vi "closetiffs.vi"   [LabVIEW 2015]
types:
  T1 = typedef "LVRectTypeDef.ctl" = cluster{"Left":i16, "Top":i16, "Right":i16, "Bottom":i16}
  T2 = cluster{"Xpixels":i32, "Vxminref":dbl, "Vxmaxref":dbl, "P":dbl, "Ypixels":i32, "Vyminref":dbl, "Vymaxref":dbl, "srate":sgl, "sAOxy":i32, "timeout":dbl, "type":string, "date":string, "time":string, "Colormap":u16, "Drawing Mode":u16, "Scanning Mode":u16, "square pixels":bool, "square matrix":bool, "Xpixels Img":i32, "Vx-min Img":dbl, "VX-max Img":dbl, "Ypixels Img":i32, "Vy-min Img":dbl, "Vy-max Img ":dbl, "Angle Img":dbl, "autoshutter":bool, "finite":bool, "cont":bool, "wavdet":bool, "measpoints":i32, "avpp":i32, "bufferAO":i32, "bufferAI":i32, "starttick":u32, "waveform":path, "Vx-ref":dbl, "Vy-ref":dbl, "refreshrate":dbl, "refreshbuffer":i32, "tt_cycles":i32, "motorref":refnum<k7>, "mirrorswitch":refnum<k7>, "sample mode":i32, "maxbufferAI":i32, "srateAODO":sgl, "bin":sgl, "Pel":sgl, "Angle draw":dbl, "srate Img":sgl, "ROIimg_plotbounds":T1, "auto OD":bool, "ODfilt":u16, "aAI":i32[], "aCI":i32[], "aAO":u32[], "aDO":u32[], "refwfsize":dbl, "Lifetime":bool, "Vz-Img":dbl, "Vz-ref":dbl, "Vz-reset":dbl, "AIoverride":bool, "aAS":u32[], "XYZstart":dbl[], "External 100KHz Clock?":bool}
  T3 = cluster{"filetif":refnum<file>[], "E_filetif":errorcluster[]}
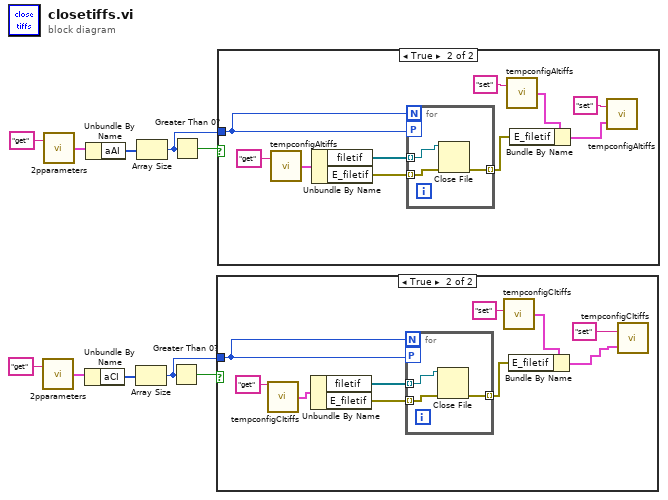
[diagram p0: block diagram]
diagram:
  n1 = call "2pparameters.vi"("command"="get") -> ("params out"=w1:T2)  [unwired: 1 in]
  n2 = call "2pparameters.vi"("command"="get") -> ("params out"=w10:T2)  [unwired: 1 in]
  n3 = Unbundle By Name(w1) -> ("aCI"=w3:i32[])
  n4 = Unbundle By Name(w10) -> ("aAI"=w8:i32[])
  n5 = Array Size(array=w3) -> (size(s)=w5:i32)
  n6 = Array Size(array=w8) -> (size(s)=w6:i32)
  n7 = Greater Than 0?(x=w5) -> (x > 0?=w4:bool)
  n8 = Greater Than 0?(x=w6) -> (x > 0?=w7:bool)
  n9 = case shown="True" w4 {
    tunnel: w5 -> [_ w17]
    frame False {
    }
    frame True {
      n10 = call "tempconfigCItiffs.vi"("command"="get") -> ("Temp Config out"=w15:T3)  [unwired: 1 in]
      n11 = Unbundle By Name(w15) -> ("filetif"=w20:refnum<file>[], "E_filetif"=w19:errorcluster[])
      n12 = for {
        N: w17 -> [_]
        workers-P: w17 -> [_]
        tunnel: w20 -> [w23] mode=indexing
        tunnel: w19 -> [w22] mode=indexing
        tunnel: [w21] -> w18 mode=indexing
        n13 = Close File(refnum=w23, error in=w22) -> (error out=w21:errorcluster)  [unwired: 1 out]
      }
      n14 = call "tempconfigCItiffs.vi"("command"="set") -> ("Temp Config out"=w13:T3)  [unwired: 1 in]
      n15 = Bundle By Name(cluster=w13, "E_filetif"=w18) -> (w11:T3)
      n16 = call "tempconfigCItiffs.vi"("Temp Config in"=w11, "command"="set") -> ()  [unwired: 1 out]
    }
  }
  n17 = case shown="True" w7 {
    tunnel: w6 -> [_ w24]
    frame False {
    }
    frame True {
      n18 = call "tempconfigAItiffs.vi"("command"="get") -> ("Temp Config out"=w31:T3)  [unwired: 1 in]
      n19 = Unbundle By Name(w31) -> ("filetif"=w27:refnum<file>[], "E_filetif"=w26:errorcluster[])
      n20 = for {
        N: w24 -> [_]
        workers-P: w24 -> [_]
        tunnel: w27 -> [w36] mode=indexing
        tunnel: w26 -> [w35] mode=indexing
        tunnel: [w34] -> w25 mode=indexing
        n21 = Close File(refnum=w36, error in=w35) -> (error out=w34:errorcluster)  [unwired: 1 out]
      }
      n22 = call "tempconfigAItiffs.vi"("command"="set") -> ("Temp Config out"=w30:T3)  [unwired: 1 in]
      n23 = Bundle By Name(cluster=w30, "E_filetif"=w25) -> (w28:T3)
      n24 = call "tempconfigAItiffs.vi"("Temp Config in"=w28, "command"="set") -> ()  [unwired: 1 out]
    }
  }
